vi "Build Array.vi"() -> ()   [LabVIEW 2025]
panel:
  in  "?":bool
  in  "Index":i32
  in  "?":bool
  out "Output Array":dbl[](array[numeric])
  in  "Element to Insert":dbl
  # "ME 235: Design of Microprocessor Based Mechanical Systems"
  # "Lab 2 - Build Arrray"
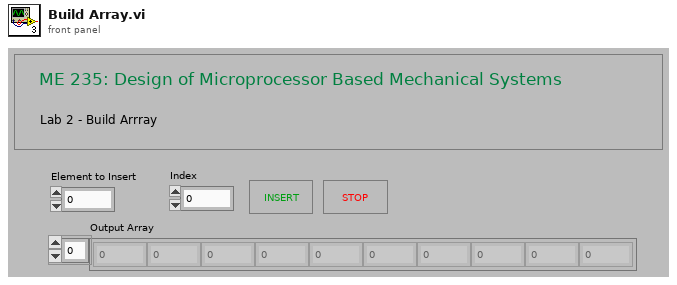
[diagram p1: front panel]
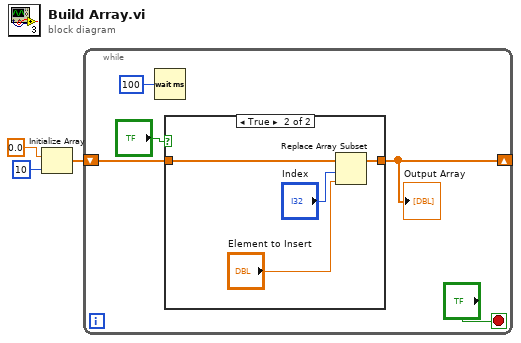
[diagram p0: block diagram]
diagram:
  n1 = Initialize Array(0.0, 10) -> (w1:dbl[])
  n2 = while {
    shift-right: [w5] -> _
    shift-left: w1 -> [w6]
    stop <- "?" stop-if-true
    n3 = Wait (ms)(milliseconds to wait=u32 100) -> ()  [unwired: 1 out]
    n4 = case shown="True" "?" {
      tunnel: w6 -> [w9 w11]
      tunnel: [w9 w10] -> w5
      frame False {
      }
      frame True {
        n5 = Replace Array Subset(array=w11, new element="Element to Insert", index="Index") -> (w10:dbl[])
      }
    }
    "Output Array" <- w5
  }
